vi "Laser_Startup_Burst.vi"(1 "Error In":errorcluster) -> (0 "Lambda":dbl, 2 "Error Out":errorcluster)   [LabVIEW 2016]
uses:
  Utility/Global_Laser.vi
  Program Files (x86)/OPOTEK_DLL/OPOTEK.dll
panel:
  out "error_Code":i32
  out "laserCOMPort":i32
  out "motorCOMPort":i32
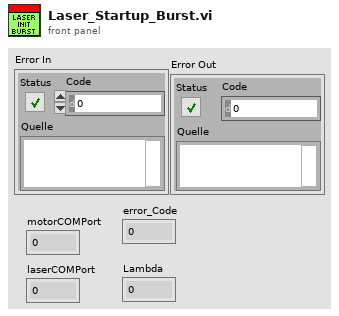
[diagram p1: front panel]
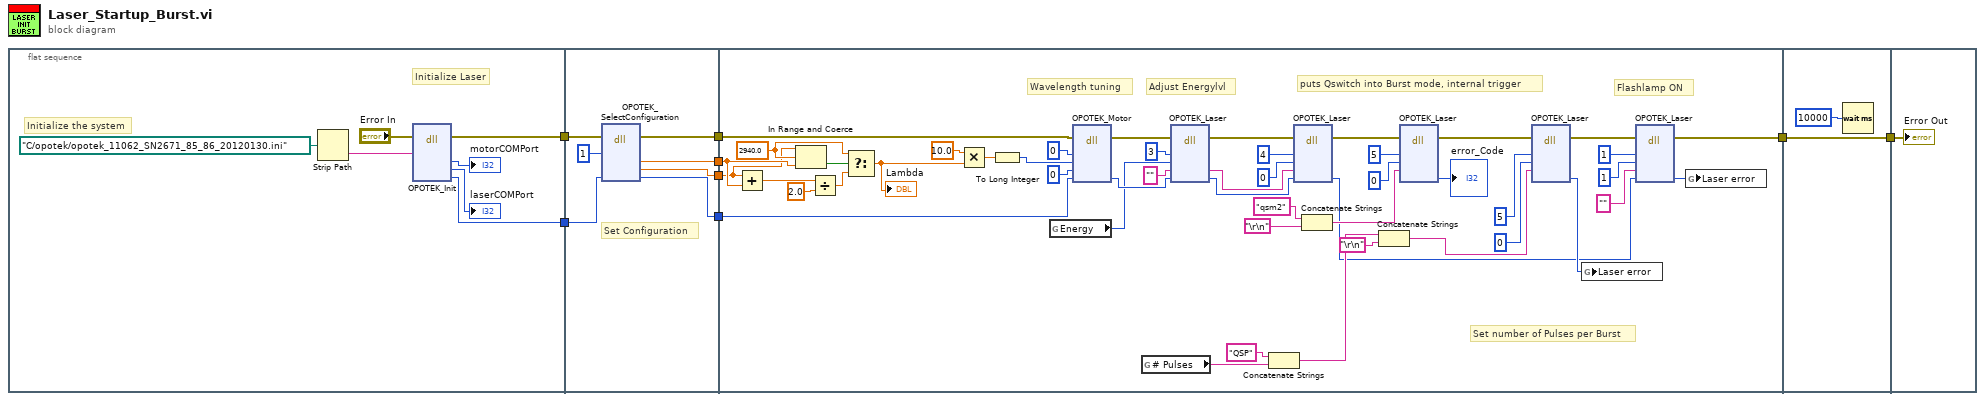
[diagram p0: block diagram]
diagram:
  n1 = flat-sequence {
    tunnel: [w10] -> w8
    tunnel: [w9] -> w2
    tunnel: w8 -> [w17]
    tunnel: [w19] -> w7
    tunnel: [w20] -> w6
    tunnel: [w16] -> w5
    tunnel: w2 -> [w21]
    tunnel: [w18] -> w1
    tunnel: w7 -> [w65]
    tunnel: w6 -> [w64]
    tunnel: w5 -> [w56]
    tunnel: [w49] -> w4
    tunnel: w1 -> [w57]
    tunnel: w4 -> [w71]
    tunnel: [w71] -> w3
    tunnel: w3 -> [w73]
    frame #0 {
      # "Initialize Laser"
      # "Initialize the system"
      n2 = Strip Path(path=path "C:/opotek/opotek_11062_SN2671_85_86_20120130.ini" ("Pfad")) -> (name=w11:string)  [unwired: 1 out]
      n3 = dll-call lib="C:/Program Files (x86)/OPOTEK_DLL/OPOTEK.dll" fn="OPOTEK_Init"(error in="Error In", "INI_File"=w11) -> (error out=w10:errorcluster, "motorCOMPort"=→"motorCOMPort":i32, "laserCOMPort"=→"laserCOMPort":i32, "error_Code"=w9:i32)  [unwired: 7 in, 1 out]
    }
    frame #1 {
      # "Set Configuration"
      n4 = dll-call lib="C:/Program Files (x86)/OPOTEK_DLL/OPOTEK.dll" fn="OPOTEK_SelectConfiguration"(error in=w17, "configuration"=u8 1, "error_Code"=w21) -> (error out=w16:errorcluster, "wavelength_Low"=w19:dbl, "wavelength_High"=w20:dbl, "error_Code"=w18:i32)  [unwired: 6 in, 1 out]
    }
    frame #2 {
      w67 = 2940.0 ("Wavelength (nm)")
      # "Set number of Pulses per Burst"
      # "puts Qswitch into Burst mode, internal trigger"
      # "Flashlamp ON"
      # "Adjust Energylvl"
      # "Wavelength tuning"
      n5 = Add(x=w64, y=w65) -> (x+y=w68:dbl)
      n6 = In Range and Coerce(upper limit=w64, x=w67, lower limit=w65) -> (In Range?=w66:bool)  [unwired: 1 out]
      n7 = Divide(x=w68, y=2.0) -> (x/y=w70:dbl)
      n8 = Select(t=w67, s=w66, f=w70) -> (s? t:f=w58:dbl)
      "Lambda" <- w58
      n9 = Multiply(x=10.0, y=w58) -> (x*y=w61:dbl)
      n10 = To Long Integer(number=w61) -> (32bit integer=w62:i32)
      n11 = global read "Global_Laser.vi" "Energy"() -> (w48:i16)
      n12 = dll-call lib="C:/Program Files (x86)/OPOTEK_DLL/OPOTEK.dll" fn="OPOTEK_Motor"(error in=w56, "action"=i8 0, "parameter1"=w62, "parameter2"=0, "error_Code"=w57) -> (error out=w53:errorcluster, "error_Code"=w54:i32)  [unwired: 6 in, 1 out]
      n13 = global read "Global_Laser.vi" "# Pulses"() -> (w45:string)
      n14 = dll-call lib="C:/Program Files (x86)/OPOTEK_DLL/OPOTEK.dll" fn="OPOTEK_Laser"(error in=w53, "action"=i8 3, "parameter"=w48, "stringToSend"="", "error_Code"=w54) -> (error out=w27:errorcluster, "stringToSend"=w29:string, "error_Code"=w25:i32)  [unwired: 5 in, 1 out]
      n15 = Concatenate Strings("QSP", w45) -> (w43:string)
      n16 = dll-call lib="C:/Program Files (x86)/OPOTEK_DLL/OPOTEK.dll" fn="OPOTEK_Laser"(error in=w27, "action"=i8 4, "parameter"=i16 0, "stringToSend"=w29, "error_Code"=w25) -> (error out=w28:errorcluster, "error_Code"=w24:i32)  [unwired: 6 in, 1 out]
      n17 = Concatenate Strings("qsm2" ("String"), "\r\n") -> (w31:string)
      n18 = Concatenate Strings(w43, "\r\n") -> (w44:string)
      n19 = dll-call lib="C:/Program Files (x86)/OPOTEK_DLL/OPOTEK.dll" fn="OPOTEK_Laser"(error in=w28, "action"=i8 5, "parameter"=i16 0, "stringToSend"=w31) -> (error out=w38:errorcluster, "error_Code"=→"error_Code":i32)  [unwired: 7 in, 1 out]
      n20 = dll-call lib="C:/Program Files (x86)/OPOTEK_DLL/OPOTEK.dll" fn="OPOTEK_Laser"(error in=w38, "action"=i8 5, "parameter"=i16 0, "stringToSend"=w44) -> (error out=w30:errorcluster, "error_Code"=w37:i32)  [unwired: 7 in, 1 out]
      n21 = global write "Global_Laser.vi" "Laser error"(w37) -> ()
      n22 = dll-call lib="C:/Program Files (x86)/OPOTEK_DLL/OPOTEK.dll" fn="OPOTEK_Laser"(error in=w30, "action"=i8 1, "parameter"=i16 1, "stringToSend"="", "error_Code"=w24) -> (error out=w49:errorcluster, "error_Code"=w47:i32)  [unwired: 6 in, 1 out]
      n23 = global write "Global_Laser.vi" "Laser error"(w47) -> ()
    }
    frame #3 {
      n24 = Wait (ms)(milliseconds to wait=u32 10000) -> ()  [unwired: 1 out]
    }
    frame #4 {
      "Error Out" <- w73
    }
  }
